vi "SlopeAndInterceptFromPoints (SubVI).vi"(11 "Array (stage frame, mm)":dbl[][][](array[numeric])) -> (0 "all intercepts":dbl[][](array[numeric]), 3 "all slopes":dbl[](array[numeric]))   [LabVIEW 2016]
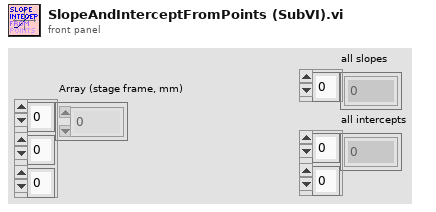
[diagram p1: front panel]
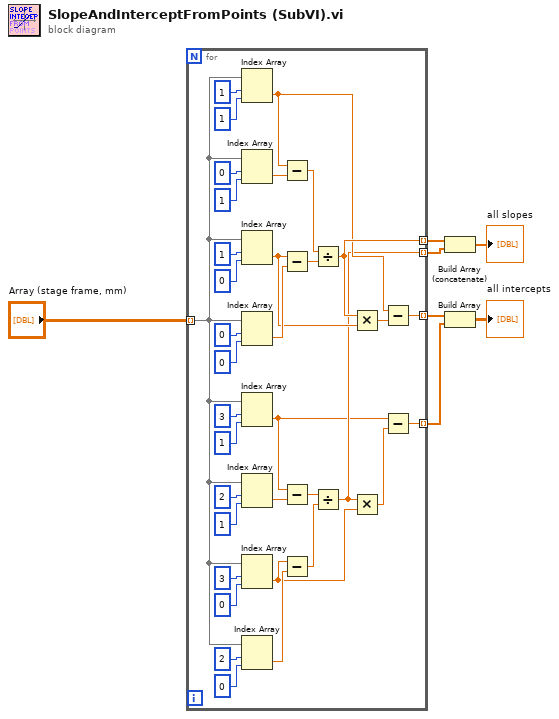
[diagram p0: block diagram]
diagram:
  n1 = for {
    tunnel: "Array (stage frame, mm)" -> [w18] mode=indexing
    tunnel: [w17] -> w5 mode=indexing
    tunnel: [w12] -> w6 mode=indexing
    tunnel: [w13] -> w2 mode=indexing
    tunnel: [w8] -> w3 mode=indexing
    n2 = Index Array(array=w18, index (row)=1 ("disabled index (row)"), index (col)=1 ("disabled index (col)")) -> (element=w15:dbl)
    n3 = Index Array(array=w18, index (row)=0 ("disabled index (row)"), index (col)=1 ("disabled index (col)")) -> (element=w40:dbl)
    n4 = Index Array(array=w18, index (row)=1 ("disabled index (row)"), index (col)=0 ("disabled index (col)")) -> (element=w16:dbl)
    n5 = Index Array(array=w18, index (row)=0 ("disabled index (row)"), index (col)=0 ("disabled index (col)")) -> (element=w36:dbl)
    n6 = Index Array(array=w18, index (row)=3 ("disabled index (row)"), index (col)=1 ("disabled index (col)")) -> (element=w9:dbl)
    n7 = Index Array(array=w18, index (row)=2 ("disabled index (row)"), index (col)=1 ("disabled index (col)")) -> (element=w28:dbl)
    n8 = Index Array(array=w18, index (row)=3 ("disabled index (row)"), index (col)=0 ("disabled index (col)")) -> (element=w11:dbl)
    n9 = Index Array(array=w18, index (row)=2 ("disabled index (row)"), index (col)=0 ("disabled index (col)")) -> (element=w24:dbl)
    n10 = Subtract(x=w15, y=w40) -> (x-y=w39:dbl)
    n11 = Subtract(x=w16, y=w36) -> (x-y=w35:dbl)
    n12 = Subtract(x=w9, y=w28) -> (x-y=w27:dbl)
    n13 = Subtract(x=w11, y=w24) -> (x-y=w23:dbl)
    n14 = Divide(x=w39, y=w35) -> (x/y=w17:dbl)
    n15 = Divide(x=w27, y=w23) -> (x/y=w12:dbl)
    n16 = Multiply(x=w17, y=w16) -> (x*y=w14:dbl)
    n17 = Multiply(x=w12, y=w11) -> (x*y=w10:dbl)
    n18 = Subtract(x=w15, y=w14) -> (x-y=w13:dbl)
    n19 = Subtract(x=w9, y=w10) -> (x-y=w8:dbl)
  }
  n20 = Build Array (concatenate)(w5, w6) -> (→"all slopes":dbl[])
  n21 = Build Array(w2, w3) -> (→"all intercepts":dbl[][])
